vi "configDAQmx.AI.vi"(8 "error in (no error)":errorcluster, 9 "DAQmx.AI.config":T1={"AI.Coupling"=10045, "input terminal configuration "=-1} {"input terminal configuration" items=["default"=-1, "RSE"=10083, "NRSE"=10078, "Differential"=10106, "Pseudodifferential"=12529]; "AI.Coupling" items=["AC"=10045, "DC"=10050, "GND"=10066]}, 10 "DAQ.config":T2={"Channels"="", "DAQ_Type"=enum."AI", "minimum value"=-5.0, "maximum value"=5.0, "DAQ_SamplingInfo"={"Fs"=0.0, "#s"=0.0}, "DAQ_SamplingMode"=enum."Continuous"} {"maximum value" format="%0.2f"; "minimum value" format="%0.2f"}, 11 "DAQmx.AI in":refnum<class "DAQmx.AI.lvclass">) -> (0 "error out":errorcluster, 3 "DAQmx.AI out":refnum<class "DAQmx.AI.lvclass">)   [LabVIEW 2016, in "DAQmx.AI.lvclass"]
uses:
  DAQmx.AI.lvclass
  C:/user/patrick/hg/lockin.SMO/lvsrc/SMOs/DAQmx/DAQmx.lvclass
  DAQ/Typedefs/DAQ_Config.ctl
  DAQ/Typedefs/PrivateEvents--DAQ.AI.Channels.ctl
  DAQ/Typedefs/DAQ_Type.ctl
  DAQ/Typedefs/DAQ_SamplingInfo.ctl
  DAQ/Typedefs/DAQ_SamplingMode.ctl
  Typedefs/DAQmx.AI_Config.ctl
  DAQmx.AI.lvclass/DAQmx.AI.ctl
  DAQmx/DAQmx.lvclass
  DAQ/DAQ.lvclass
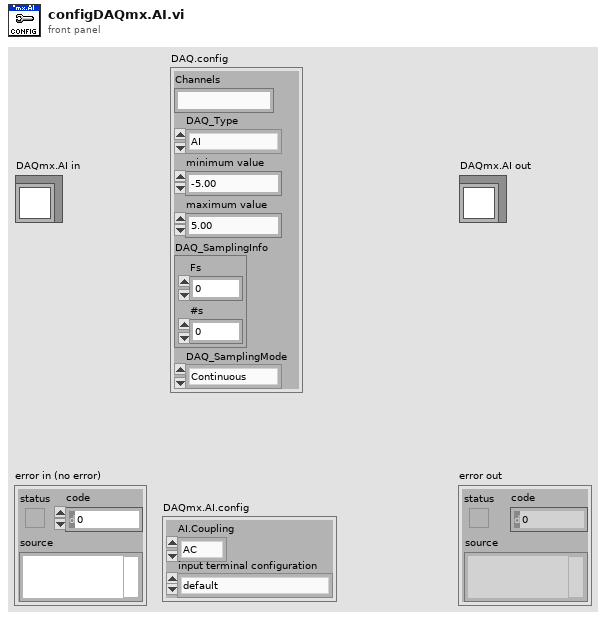
[diagram p1: front panel]
types:
  T1 = typedef "DAQmx.AI.lvclass/DAQmx.AI_Config.ctl" = cluster{"AI.Coupling":i32, "input terminal configuration ":i32}
  T2 = typedef "DAQ.lvclass/DAQ_Config.ctl" = cluster{"Channels":T3, "DAQ_Type":T4, "minimum value":dbl, "maximum value":dbl, "DAQ_SamplingInfo":T5, "DAQ_SamplingMode":T6}
  T3 = typedef "DAQ.lvclass/PrivateEvents--DAQ.AI.Channels.ctl" = string
  T4 = typedef "DAQ.lvclass/DAQ_Type.ctl" = enum16{"AI", "AO"}
  T5 = typedef "DAQ.lvclass/DAQ_SamplingInfo.ctl" = cluster{"Fs":dbl, "#s":dbl}
  T6 = typedef "DAQ.lvclass/DAQ_SamplingMode.ctl" = enum16{"Continuous", "Finite"}
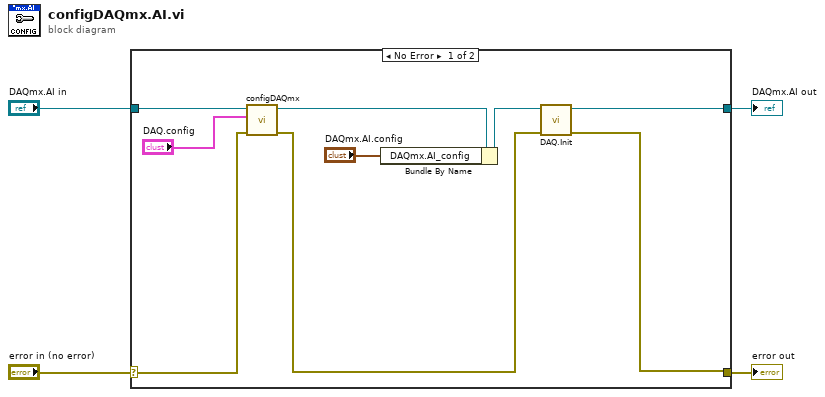
[diagram p0: block diagram]
diagram:
  n1 = case shown="No Error" "error in (no error)" {
    selector: "error in (no error)" -> [w8 w15]
    tunnel: [w6 w15] -> w3
    tunnel: [w5 w14] -> w1
    tunnel: "DAQmx.AI in" -> [w12 w14]
    frame No Error {
      n2 = call "configDAQmx.vi"("error in (no error)"=w8, "DAQ.Config"="DAQ.config", "DAQmx in"=w12) -> ("error out"=w7:errorcluster, "DAQmx out"=w11:refnum<class "DAQmx.AI.lvclass">)  [unwired: 7 in]
      n3 = Bundle By Name(cluster=w11, "DAQmx.AI_config"="DAQmx.AI.config") -> (w9:refnum<class "DAQmx.AI.lvclass">)
      n4 = call-dynamic "DAQ.Init.vi"("error in (no error)"=w7, "DAQmx.AI in"=w9) -> ("error out"=w6:errorcluster, "DAQmx.AI out"=w5:refnum<class "DAQmx.AI.lvclass">)  [unwired: 8 in]
    }
    frame Error {
    }
  }
  "error out" <- w3
  "DAQmx.AI out" <- w1
